vi "Movimiento.vi"() -> ()   [LabVIEW 2018]
uses:
  <vilib>/Motion/Express/_s/nimc.fb.straightLineMove.startStraightLineMove.axis.modeRelative.0.vi
  <vilib>/Motion/BlockNode/FB.NIMotion.xnode
  <vilib>/functionblocks/FB Property/FB Overlay DBL.ctl
panel:
  in  "start":bool
  in  "3a 3":bool
  in  "2a 3":bool
  in  "1a 3":bool
  in  "3a 2":bool
  in  "2a 2":bool
  in  "1a 2":bool
  out "Enum":T1(ring)
  in  "3a":bool
  in  "2a":bool
  in  "1a":bool
  out "Done2":bool
  in  "Izquieda":bool
  in  "Derecha":bool
  in  "Rojo":bool
  in  "Amarillo":bool
  in  "Azul":bool
  in  "Verde":bool
  in  "stop":bool
  out "Done3":bool
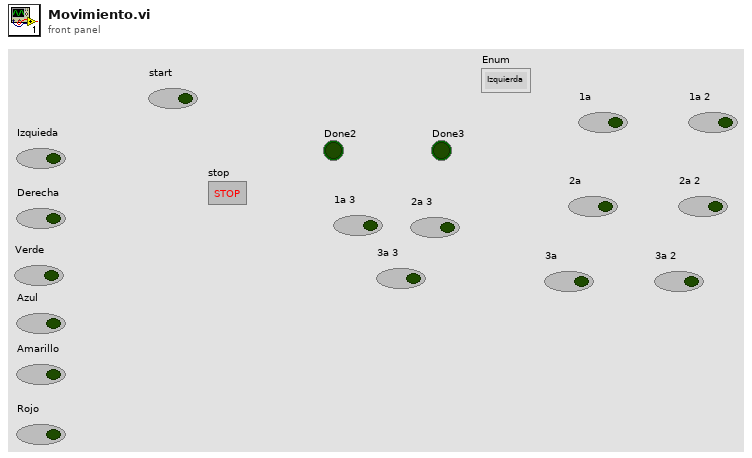
[diagram p1: front panel]
types:
  T1 = enum16{"Izquierda", "Centro", "Derecha", "izq2", "cent2", "der2", "izq3", "cent3", "der3"}
  T2 = enum16{"Izquierda", "Centro", "Derecha", "izq2", "cent2", "der2", "izq3", "cent3", "der3", "inicio", "Inicio2"}
  T3 = enum16{"Izquierda", "Centro", "Derecha", "izq2", "cent2", "der2", "izq3", "cent3", "der3", "inicio"}
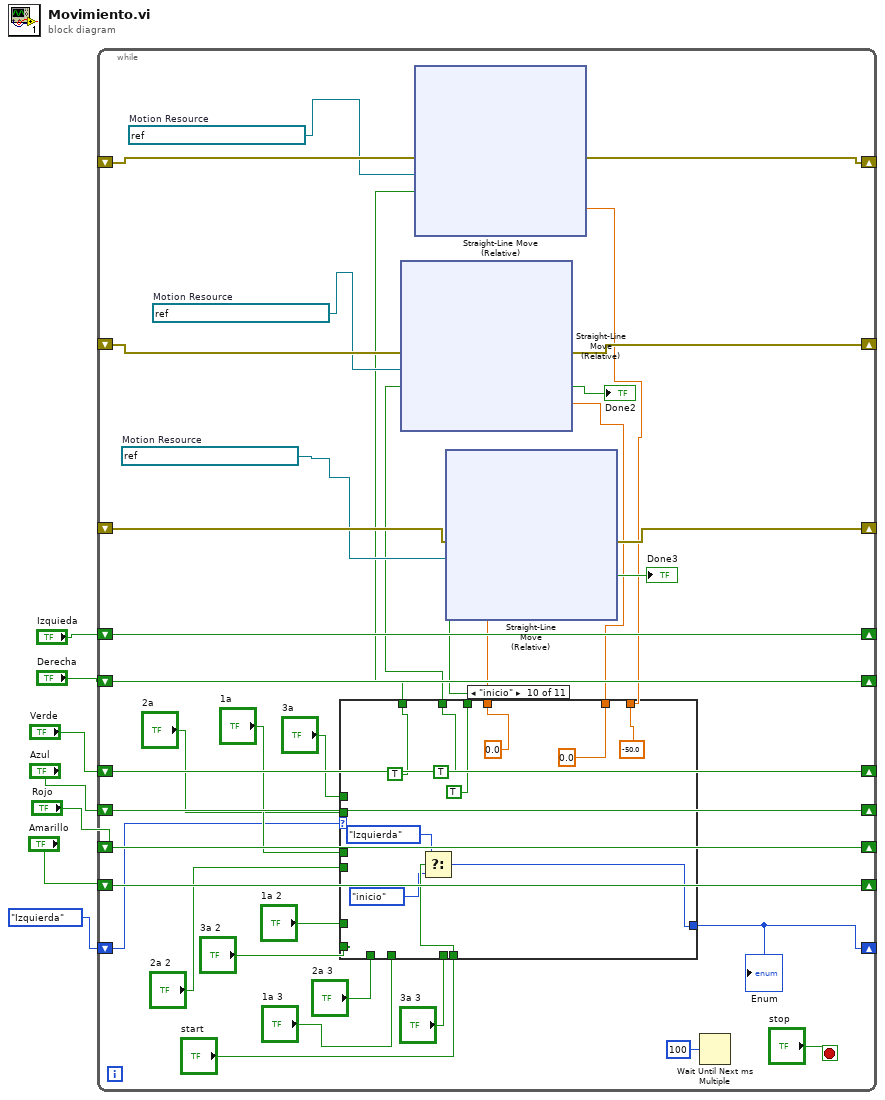
[diagram p0: block diagram]
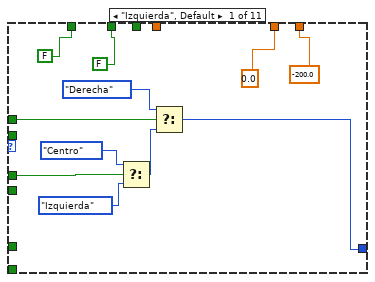
[diagram p2: hidden frame]
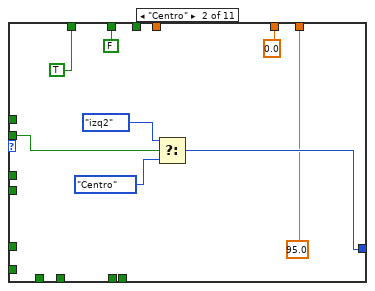
[diagram p3: hidden frame]
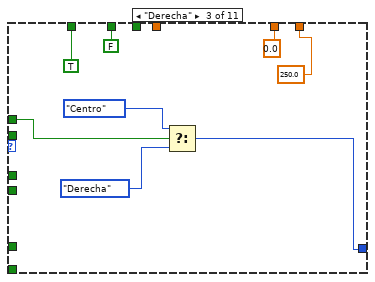
[diagram p4: hidden frame]
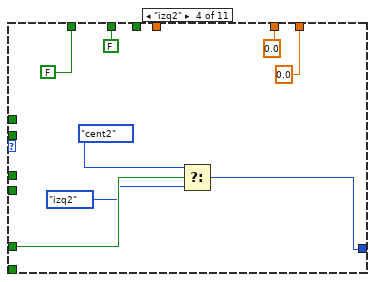
[diagram p5: hidden frame]
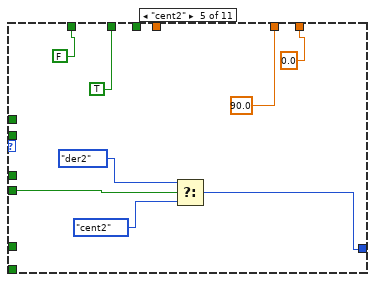
[diagram p6: hidden frame]
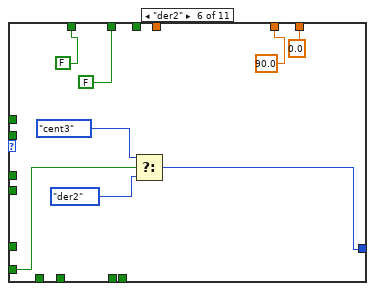
[diagram p7: hidden frame]
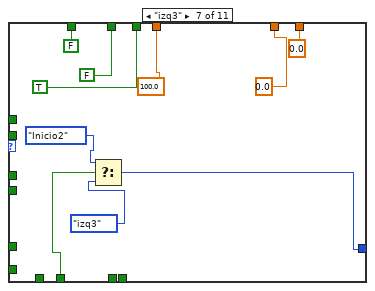
[diagram p8: hidden frame]
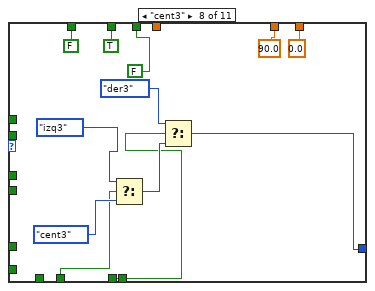
[diagram p9: hidden frame]
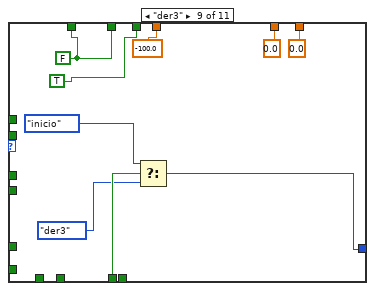
[diagram p10: hidden frame]
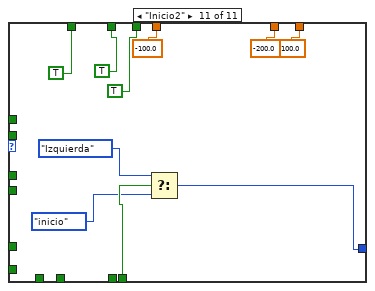
[diagram p11: hidden frame]
diagram:
  n1 = while {
    shift-right: [w41] -> _
    shift-left: _ -> [w42]
    shift-right: [w36] -> _
    shift-left: _ -> [w35]
    shift-right: [w37] -> _
    shift-left: _ -> [w38]
    shift-right: [w30] -> _
    shift-left: "Verde" -> [w30]
    shift-right: [w31] -> _
    shift-left: "Azul" -> [w31]
    shift-right: [w32] -> _
    shift-left: "Rojo" -> [w32]
    shift-right: [w33] -> _
    shift-left: "Amarillo" -> [w33]
    shift-right: [w34] -> _
    shift-left: "Izquieda" -> [w34]
    shift-right: [w29] -> _
    shift-left: "Derecha" -> [w29]
    shift-right: [w22] -> _
    shift-left: T2."Izquierda" -> [w23]
    stop <- "stop" stop-if-true
    w26 = refnum<k21> "nism://My Computer/Axis 3"  # Motion Resource
    w27 = refnum<k21> "nism://My Computer/Axis 2"  # Motion Resource
    w28 = refnum<k21> "nism://My Computer/Axis 1"  # Motion Resource
    n2 = case shown="\"inicio\"" w23 {
      tunnel: "3a" -> [w54 _ w71 _ _ _ _ _ _ _ _]
      tunnel: "1a" -> [w53 _ _ _ _ _ _ _ _ _ _]
      tunnel: [w49 w60 w68 w76 w84 w88 w99 w112 w118 w127 w137] -> w22
      tunnel: "2a" -> [_ w63 _ _ _ _ _ _ _ _ _]
      tunnel: [-200.0 95.0 250.0 0.0 0.0 0.0 0.0 0.0 0.0 -50.0 -100.0] -> w20
      tunnel: [FALSE TRUE TRUE FALSE FALSE FALSE FALSE FALSE w122 TRUE TRUE] -> w19
      tunnel: "1a 2" -> [_ _ _ w79 _ _ _ _ _ _ _]
      tunnel: "3a 2" -> [_ _ _ _ _ w91 _ _ _ _ _]
      tunnel: "2a 2" -> [_ _ _ _ w87 _ _ _ _ _ _]
      tunnel: [FALSE FALSE FALSE FALSE TRUE FALSE FALSE TRUE w122 TRUE TRUE] -> w15
      tunnel: [0.0 0.0 0.0 0.0 90.0 90.0 0.0 90.0 0.0 0.0 -200.0] -> w14
      tunnel: "2a 3" -> [_ _ _ _ _ _ _ _ _ _ _]
      tunnel: "1a 3" -> [_ _ _ _ _ _ w97 w106 _ _ _]
      tunnel: "3a 3" -> [_ _ _ _ _ _ _ w116 w121 _ _]
      tunnel: [_ _ _ _ _ _ 100.0 _ -100.0 0.0 -100.0] -> w10
      tunnel: [_ _ _ _ _ _ TRUE FALSE TRUE TRUE TRUE] -> w9
      tunnel: "start" -> [_ _ _ _ _ _ _ _ _ w130 w140]
      frame "Izquierda", Default {
        n3 = Select(t=T1."Centro", s=w53, f=T1."Izquierda") -> (s? t:f=w55:T1)
        n4 = Select(t=T1."Derecha", s=w54, f=w55) -> (s? t:f=w49:T1)
      }
      frame "Centro" {
        n5 = Select(t=T1."izq2", s=w63, f=T1."Centro") -> (s? t:f=w60:T1)
      }
      frame "Derecha" {
        n6 = Select(t=T1."Centro", s=w71, f=T1."Derecha") -> (s? t:f=w68:T1)
      }
      frame "izq2" {
        n7 = Select(t=T1."cent2", s=w79, f=T1."izq2") -> (s? t:f=w76:T1)
      }
      frame "cent2" {
        n8 = Select(t=T1."der2", s=w87, f=T1."cent2") -> (s? t:f=w84:T1)
      }
      frame "der2" {
        n9 = Select(t=T1."cent3", s=w91, f=T1."der2") -> (s? t:f=w88:T1)
      }
      frame "izq3" {
        n10 = Select(t=T2."Inicio2", s=w97, f=T2."izq3") -> (s? t:f=w99:T2)
      }
      frame "cent3" {
        n11 = Select(t=T1."izq3", s=w106, f=T1."cent3") -> (s? t:f=w117:T1)
        n12 = Select(t=T1."der3", s=w116, f=w117) -> (s? t:f=w112:T1)
      }
      frame "der3" {
        w122 = FALSE
        n13 = Select(t=T3."inicio", s=w121, f=T3."der3") -> (s? t:f=w118:T3)
      }
      frame "inicio" {
        n14 = Select(t=T2."Izquierda", s=w130, f=T2."inicio") -> (s? t:f=w127:T2)
      }
      frame "Inicio2" {
        n15 = Select(t=T3."Izquierda", s=w140, f=T3."inicio") -> (s? t:f=w137:T3)
      }
    }
    "Enum" <- w22
    n16 = xnode "Straight-Line Move\n(Relative)"("error in"=w38, "resource"=w27, "execute"=w15, "position"=w14) -> ("error out"=w37:errorcluster, "done"=→"Done2":bool)  [unwired: 1 out]
    n17 = xnode "Straight-Line Move\n(Relative)"("error in"=w35, "resource"=w28, "execute"=w19, "position"=w20) -> ("error out"=w36:errorcluster)  [unwired: 2 out]
    n18 = xnode "Straight-Line Move\n(Relative)"("error in"=w42, "resource"=w26, "execute"=w9, "position"=w10) -> ("error out"=w41:errorcluster, "done"=→"Done3":bool)  [unwired: 1 out]
    n19 = Wait Until Next ms Multiple(millisecond multiple=u32 100) -> ()  [unwired: 1 out]
  }
